vi "Broadcast IODevInfo.vi"(8 "error in (no error)":errorcluster, 11 "IO Device in":refnum<class "IO Device.lvclass">) -> (0 "error out":errorcluster, 3 "IO Device out":refnum<class "IO Device.lvclass">)   [LabVIEW 2015, in "IO Device.lvlib" / "IO Device.lvclass"]
uses:
  IO Device.lvclass
  <vilib>/ActorFramework/Actor/Actor.lvclass/Actor.ctl
  IO Device.lvclass/IO Device.ctl
  <vilib>/ActorFramework/Actor/Actor.lvclass
  Sequencer/Sequencer Messages/Update IODevInfo Msg/Update IODevInfo Msg.lvclass
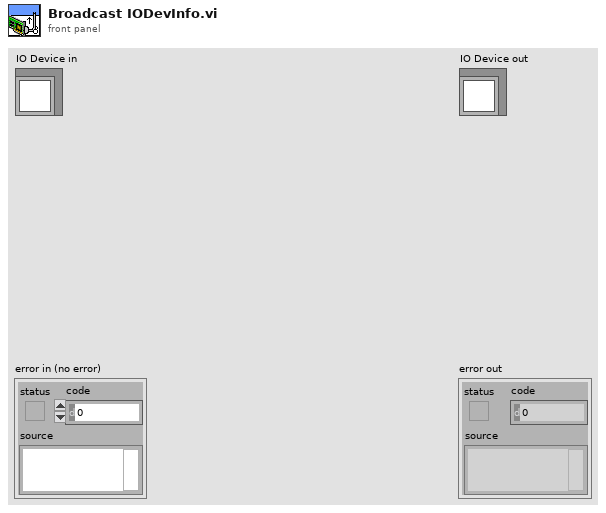
[diagram p1: front panel]
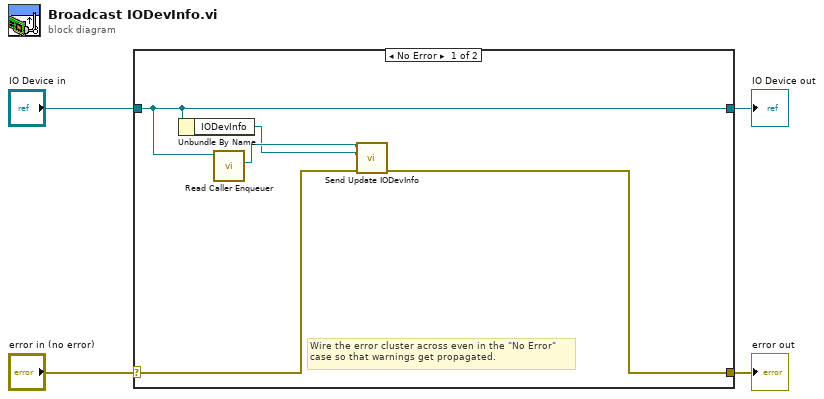
[diagram p0: block diagram]
diagram:
  n1 = case shown="No Error" "error in (no error)" {
    selector: "error in (no error)" -> [w6 w11]
    tunnel: [w5 w11] -> w3
    tunnel: [w9 w10] -> w1
    tunnel: "IO Device in" -> [w9 w10]
    frame No Error {
      # "Wire the error cluster across even in the \"No Error\"\ncase so that warnings get propagated."
      n2 = Unbundle By Name(w9) -> ("IODevInfo"=w7:refnum<class "IODevInfo.lvclass">)
      n3 = call <vilib>:"Read Caller Enqueuer.vi"("Actor"=w9) -> ("Caller Enqueuer"=w8:refnum<class "Message Enqueuer.lvclass">)  [unwired: 10 in]
      n4 = call "Send Update IODevInfo.vi"("error in (no error)"=w6, "IODevInfo"=w7, "Message Enqueuer in"=w8) -> ("error out"=w5:errorcluster)  [unwired: 7 in, 1 out]
    }
    frame Error {
    }
  }
  "error out" <- w3
  "IO Device out" <- w1
